vi "Global.vi"() -> ()   [LabVIEW 2013]
panel:
  in  "Stop":bool
  in  "DC Offset":dbl
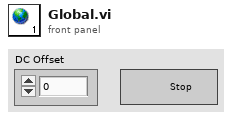
[diagram p1: front panel]
diagram:
